vi "Settings-SH.vi"(8 "Error In":errorcluster) -> (0 "error out":errorcluster, 1 "Time Target (sec)":dbl, 2 "Task":string, 3 "Subject":string)   [LabVIEW 2020, in "CollectionSupport.lvlib"]
uses:
  CollectionSupport.lvlib
panel:
  in  "Time Target (sec)":dbl
  in  "OK Button":bool
  in  "Task":string
  in  "Subject":string
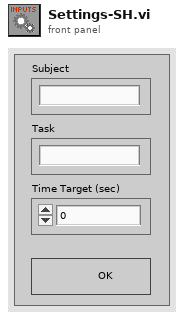
[diagram p1: front panel]
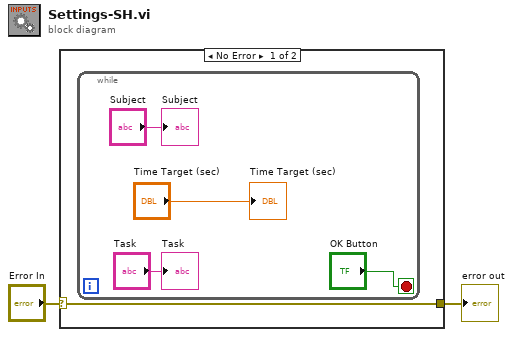
[diagram p0: block diagram]
diagram:
  n1 = case shown="No Error" "Error In" {
    selector: "Error In" -> [w3 w8]
    tunnel: [w3 w8] -> w1
    frame No Error {
      n2 = while {
        stop <- "OK Button" stop-if-true
        "Subject" <- "Subject"
        "Task" <- "Task"
        "Time Target (sec)" <- "Time Target (sec)"
      }
    }
    frame Error {
    }
  }
  "error out" <- w1
